vi "Vacuum Switch Panel.vi"() -> ()   [LabVIEW 2021]
uses:
  Classes/Controller/I-O/I-O.lvclass
  Classes/Controller/Controller.lvclass
panel:
  in  "Turn off all":bool
  out "error out":errorcluster
  out "Compression Sensor":bool
  out "Sensor Channel":dbl=6.0
  out "Sensor":bool
  out "sensor pin number":i32=3
  out "tray sensor":bool
  out "secondary valve sensor":bool
  out "primary valve sensor":bool
  in  "Turn on secondary vacuum":bool
  in  "turn on primary vacuum":bool
  in  "secure tray":bool
  out "Valve Channel":dbl=6.0
  in  "Type":enum16{"O ring Vac", "Baseplate Vac"}(ring)
  in  "Position":i32=1 min=1 max=4
  in  "Region":i32=1 min=1 max=4
  in  "On/Off":bool
  in  "Stop":bool
  in  "error in (no error)":errorcluster
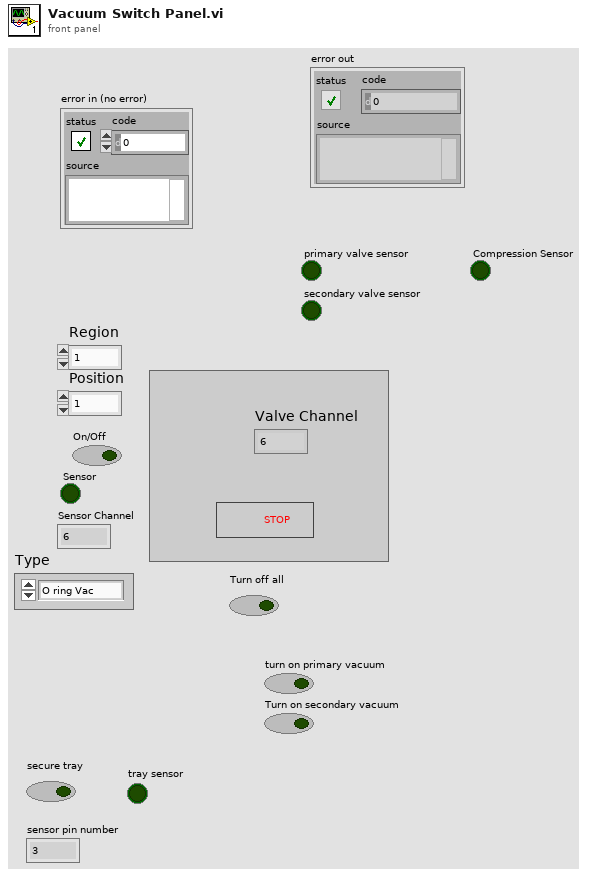
[diagram p1: front panel]
types:
  T1 = typedef "Controller.lvclass/Controllers.ctl" = cluster{"I-O.lvclass":refnum<class "I-O.lvclass">, "Gantry":refnum<k24>, "Dispenser":refnum<visa-resource-name>}
  T2 = typedef "I-O.lvclass/Pin Map.ctl" = cluster{"Region Valves":i32[], "Extra Valves":dbl[][][], "Tool Primary Valve":i32, "Tool Secondary Valve":i32, "Region Sensors":i32[], "Extra Sensors":dbl[][][], "Tool Primary Sensor":dbl, "Tool Secondary Sensor":dbl, "Compression Sensor":dbl, "5V":i32, "Dispenser Sensor":dbl, "Light Curtain":i32}
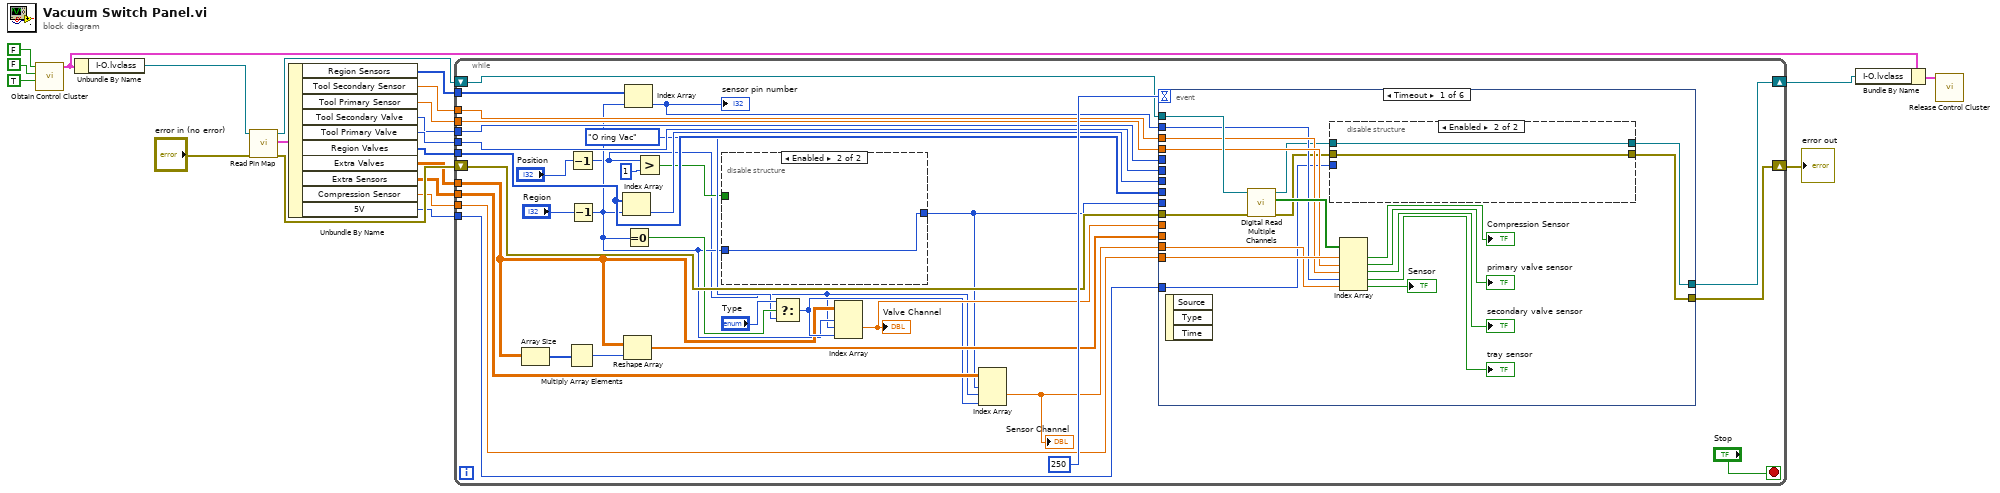
[diagram p0: block diagram]
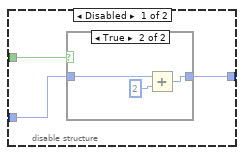
[diagram p2: hidden frame]
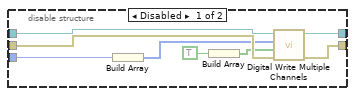
[diagram p4: hidden frame]
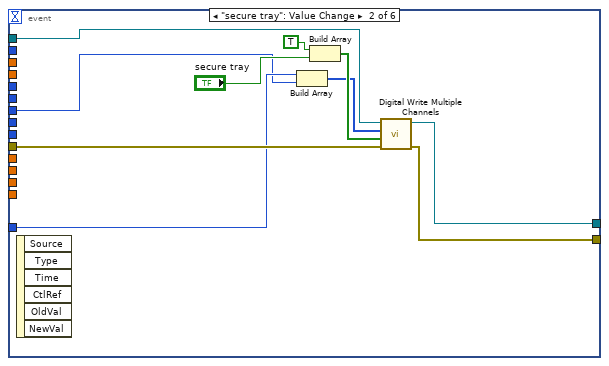
[diagram p5: hidden frame]
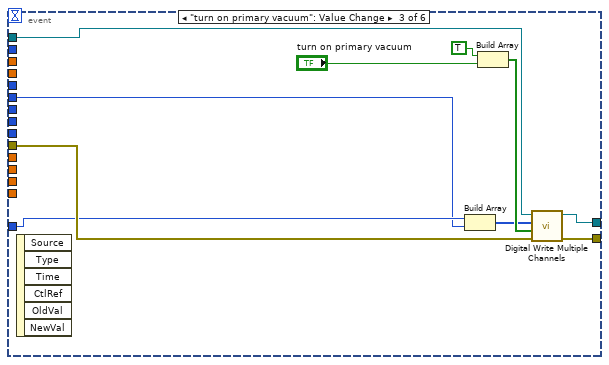
[diagram p6: hidden frame]
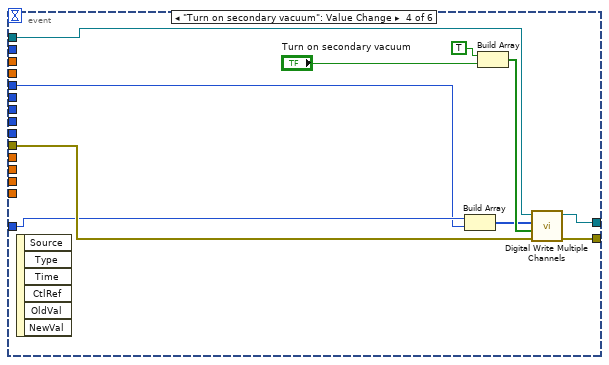
[diagram p7: hidden frame]
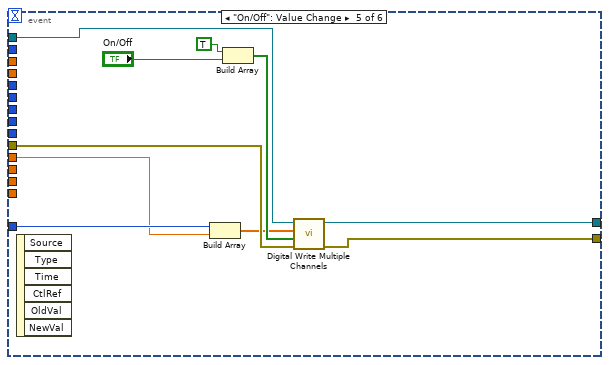
[diagram p8: hidden frame]
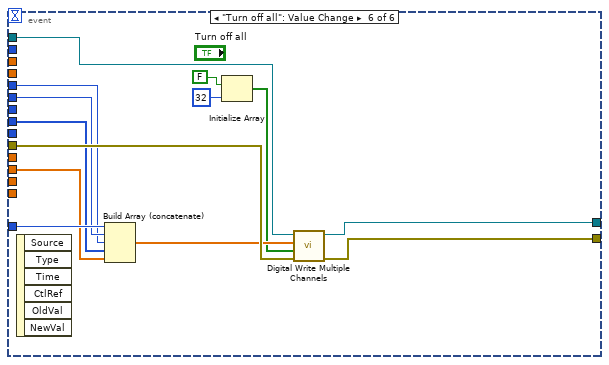
[diagram p9: hidden frame]
diagram:
  n1 = call "Obtain Control Cluster.vi"("I/O"=TRUE, "Dispense"=FALSE, "Motion"=FALSE) -> ("Control Out"=w4:T1)  [unwired: 7 in, 1 out]
  n2 = Unbundle By Name(w4) -> ("I-O.lvclass"=w18:refnum<class "I-O.lvclass">)
  n3 = call-dynamic "Read Pin Map.vi"("error in (no error)"="error in (no error)", "I-O in"=w18) -> ("error out"=w16:errorcluster, "Pin Map 2"=w22:T2, "I-O out"=w15:refnum<class "I-O.lvclass">)  [unwired: 7 in]
  n4 = Unbundle By Name(w22) -> ("Region Sensors"=w11:i32[], "Tool Secondary Sensor"=w12:dbl, "Tool Primary Sensor"=w13:dbl, "Tool Secondary Valve"=w7:i32, "Tool Primary Valve"=w8:i32, "Region Valves"=w5:i32[], "Extra Valves"=w6:dbl[][][], "Extra Sensors"=w10:dbl[][][], "Compression Sensor"=w14:dbl, "5V"=w9:i32)
  n5 = while {
    shift-right: [w53] -> w2
    shift-left: w15 -> [w54]
    shift-right: [w52] -> w1
    shift-left: w16 -> [w55]
    tunnel: w11 -> [w49]
    tunnel: w14 -> [w48]
    tunnel: w13 -> [w47]
    tunnel: w12 -> [w46]
    tunnel: w10 -> [w45]
    tunnel: w9 -> [w42]
    tunnel: w8 -> [w41]
    tunnel: w7 -> [w40]
    tunnel: w6 -> [w28]
    tunnel: w5 -> [w37]
    stop <- "Stop" stop-if-true
    n6 = Array Size(array=w28) -> (size(s)=w36:i32[])
    n7 = Multiply Array Elements(1:w36) -> (0:w35:i32)
    n8 = Decrement(x="Position") -> (x-1=w23:i32)
    n9 = Decrement(x="Region") -> (x-1=w25:i32)
    n10 = Index Array(array=w37, index=w25) -> (element=w38:i32)
    n11 = Reshape Array(w28, w35) -> (w34:dbl[])
    n12 = Index Array(array=w49, index=w25) -> (element=w44:i32)
    "sensor pin number" <- w44
    n13 = Equal To 0?(x=w25) -> (x = 0?=w32:bool)
    n14 = Greater?(x=w23, y=1) -> (0:w26:bool)
    n15 = disable-structure shown="Enabled" {
      disable-tunnel: w26 -> [w59 _]
      disable-tunnel: w25 -> [w58 w64]
      disable-tunnel: [w57 w64] -> w24
      frame Disabled {
        n16 = case shown="True" w59 {
          tunnel: w58 -> [w60 w62]
          tunnel: [w60 w61] -> w57
          frame False {
          }
          frame True {
            n17 = Add(x=w62, y=i64 2) -> (x+y=w61:i64)
          }
        }
      }
      frame Enabled {
      }
    }
    n18 = Select(t="Type", s=w32, f=enum16{"O ring Vac", "Baseplate Vac"}."O ring Vac") -> (s? t:f=w30:enum16{"O ring Vac", "Baseplate Vac"})
    n19 = Index Array(array=w28, index (dim 0)=w25, index (dim 1)=w23, index (dim 2)=w30) -> (element=w39:dbl)
    "Valve Channel" <- w39
    n20 = Index Array "Index Array"(array=w45, index (dim 0)=w24, index (dim 1)=w23, index (dim 2)=w30) -> (element=w43:dbl)
    "Sensor Channel" <- w43
    n21 = event shown="[0] Timeout" {
      selector: _ -> [_ _ _ _ _ _]
      dyn-events: _ -> [_ _ _ _ _ _]
      timeout: 250 -> [_ _ _ _ _ _]
      tunnel: w55 -> [w82 w99 w108 w120 w127 w142]
      tunnel: w54 -> [w81 w102 w112 w119 w130 w145]
      tunnel: [w68 w101 w111 w118 w129 w144] -> w53
      tunnel: [w66 w100 w107 w117 w128 w143] -> w52
      tunnel: w24 -> [_ _ _ _ _ _]
      tunnel: w48 -> [w74 _ _ _ _ _]
      tunnel: w47 -> [w73 _ _ _ _ _]
      tunnel: w46 -> [w72 _ _ _ _ _]
      tunnel: w43 -> [w71 _ _ _ _ _]
      tunnel: w44 -> [w70 _ _ _ _ _]
      tunnel: w42 -> [w65 w94 w105 w115 w125 w141]
      tunnel: w41 -> [_ _ w104 _ _ w140]
      tunnel: w40 -> [_ _ _ w114 _ w139]
      tunnel: w39 -> [_ _ _ _ w123 _]
      tunnel: w38 -> [_ w93 _ _ _ _]
      tunnel: w37 -> [_ _ _ _ _ w138]
      tunnel: w34 -> [_ _ _ _ _ w137]
      event Timeout {
        n22 = event-data() -> ()  [unwired: 1 in, 3 out]
        n23 = call-dynamic "Digital Read Multiple Channels.vi"("error in (no error)"=w82, "I-O in"=w81) -> ("error out"=w67:errorcluster, "Array 2"=w80:bool[], "I-O out"=w69:refnum<class "I-O.lvclass">)  [unwired: 7 in]
        n24 = disable-structure shown="Enabled" {
          disable-tunnel: w69 -> [w90 w92]
          disable-tunnel: [w89 w92] -> w68
          disable-tunnel: w67 -> [w88 w91]
          disable-tunnel: [w87 w91] -> w66
          disable-tunnel: w65 -> [w84 _]
          frame Disabled {
            n25 = Build Array(w84) -> (w83:i32[])
            n26 = Build Array(TRUE) -> (w86:bool[])
            n27 = call-dynamic "Digital Write Multiple Channels.vi"("error in (no error)"=w88, "values"=w86, "indices"=w83, "I-O in"=w90) -> ("error out"=w87:errorcluster, "I-O out"=w89:refnum<class "I-O.lvclass">)  [unwired: 6 in]
          }
          frame Enabled {
          }
        }
        n28 = Index Array(array=w80, index #1=w74, index #2=w73, index #3=w72, index #4=w70, index #5=w71) -> (element #1=→"Compression Sensor":bool, element #2=→"primary valve sensor":bool, element #3=→"secondary valve sensor":bool, element #4=→"tray sensor":bool, element #5=→"Sensor":bool)
      }
      event "secure tray": Value Change {
        n29 = event-data() -> ()  [unwired: 1 in, 6 out]
        n30 = Build Array(w94, w93) -> (w96:i32[])
        n31 = Build Array(TRUE ("element"), "secure tray") -> (w97:bool[])
        n32 = call-dynamic "Digital Write Multiple Channels.vi"("error in (no error)"=w99, "values"=w97, "indices"=w96, "I-O in"=w102) -> ("error out"=w100:errorcluster, "I-O out"=w101:refnum<class "I-O.lvclass">)  [unwired: 6 in]
      }
      event "turn on primary vacuum": Value Change {
        n33 = event-data() -> ()  [unwired: 1 in, 6 out]
        n34 = Build Array(w105, w104) -> (w103:i32[])
        n35 = Build Array(TRUE ("element"), "turn on primary vacuum") -> (w109:bool[])
        n36 = call-dynamic "Digital Write Multiple Channels.vi"("error in (no error)"=w108, "values"=w109, "indices"=w103, "I-O in"=w112) -> ("error out"=w107:errorcluster, "I-O out"=w111:refnum<class "I-O.lvclass">)  [unwired: 6 in]
      }
      event "Turn on secondary vacuum": Value Change {
        n37 = event-data() -> ()  [unwired: 1 in, 6 out]
        n38 = Build Array(w115, w114) -> (w113:i32[])
        n39 = Build Array(TRUE ("element"), "Turn on secondary vacuum") -> (w122:bool[])
        n40 = call-dynamic "Digital Write Multiple Channels.vi"("error in (no error)"=w120, "values"=w122, "indices"=w113, "I-O in"=w119) -> ("error out"=w117:errorcluster, "I-O out"=w118:refnum<class "I-O.lvclass">)  [unwired: 6 in]
      }
      event "On/Off": Value Change {
        n41 = event-data() -> ()  [unwired: 1 in, 6 out]
        n42 = Build Array(w125, w123) -> (w124:dbl[])
        n43 = Build Array(TRUE ("element"), "On/Off") -> (w132:bool[])
        n44 = call-dynamic "Digital Write Multiple Channels.vi"("error in (no error)"=w127, "values"=w132, "indices"=w124, "I-O in"=w130) -> ("error out"=w128:errorcluster, "I-O out"=w129:refnum<class "I-O.lvclass">)  [unwired: 6 in]
      }
      event "Turn off all": Value Change {
        n45 = event-data() -> ()  [unwired: 1 in, 6 out]
        n46 = Build Array (concatenate)(w141, w140, w139, w138, w137) -> (w136:dbl[])
        n47 = Initialize Array(FALSE, 32 ("dimension size")) -> (w133:bool[])
        n48 = call-dynamic "Digital Write Multiple Channels.vi"("error in (no error)"=w142, "values"=w133, "indices"=w136, "I-O in"=w145) -> ("error out"=w143:errorcluster, "I-O out"=w144:refnum<class "I-O.lvclass">)  [unwired: 6 in]
      }
    }
  }
  "error out" <- w1
  n49 = Bundle By Name(cluster=w4, "I-O.lvclass"=w2) -> (w3:T1)
  n50 = call "Release Control Cluster.vi"("output cluster"=w3) -> ()  [unwired: 11 in]
